vi "NicmosReadReadout.vi"(3 "refnum in":T2, 9 "error in (no error)":errorcluster) -> (0 "refnum out":T2, 2 "Readout":T1, 6 "error out":errorcluster)   [LabVIEW 2009]
uses:
  <vilib>/Utility/config.llb/Config Data RefNum.ctl
  Controls/NICMOS.READOUT.ctl
  <vilib>/Utility/config.llb/NI_LVConfig.lvlib
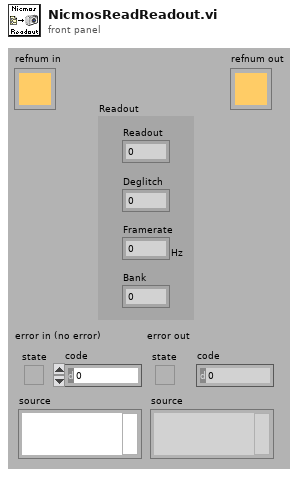
[diagram p1: front panel]
types:
  T1 = typedef "NICMOS.READOUT.ctl" = cluster{"Readout":i32, "Deglitch":i32, "Framerate":dbl[unit], "Bank":i32}
  T2 = typedef "NI_LVConfig.lvlib/Config Data RefNum.ctl" = refnum<k1>
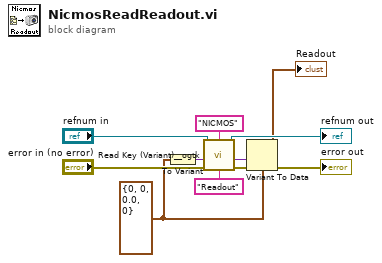
[diagram p0: block diagram]
diagram:
  w3 = T1 {"Readout"=0, "Deglitch"=0, "Framerate"=0.0, "Bank"=0} ("READOUT")
  n1 = To Variant(anything=w3) -> (Variant=w6:variant)
  n2 = call <userlib>:"Read Key (Variant)__ogtk.vi"("section"="NICMOS", "error in (no error)"="error in (no error)", "type"=w6, "key (optional)"="Readout", "refnum"="refnum in") -> ("error out"=w5:errorcluster, "key-value"=w4:variant, "refnum out"=→"refnum out":T2)  [unwired: 3 in, 1 out]
  n3 = Variant To Data(error in=w5, Variant=w4, type=w3) -> (error out=→"error out":errorcluster, data=→"Readout":T1)
